vi "Get Public Events.vi"(8 "error in (no error)":errorcluster, 11 "RPI.SenseHat.Actor in":refnum<class "RPI.SenseHat.Actor.lvclass">) -> (0 "error out":errorcluster, 2 "Public Events":T1, 3 "RPI.SenseHat.Actor out":refnum<class "RPI.SenseHat.Actor.lvclass">)   [LabVIEW 2020, in "RPI.SenseHat.Actor.lvlib" / "RPI.SenseHat.Actor.lvclass"]
uses:
  RPI.SenseHat.Actor.lvclass
  Public Events.ctl
  RPI.SenseHat.Joystick/TypeDefs/Joystick.ctl
  RPI.SenseHat.Actor.lvclass/RPI.SenseHat.Actor.ctl
  RPI.SenseHat.Joystick/RPI.SenseHat.Joystick.lvlib
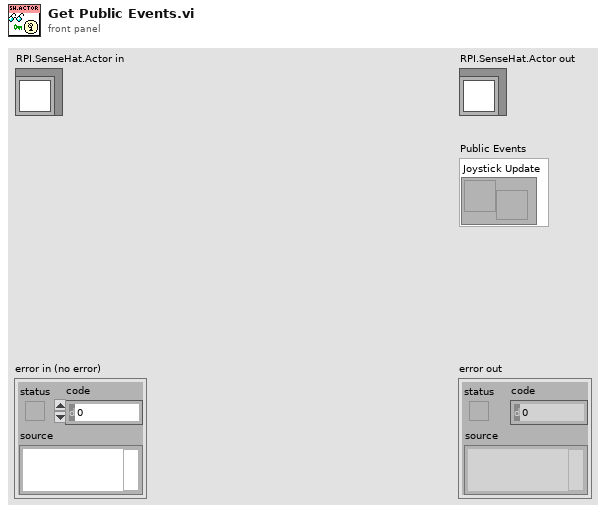
[diagram p1: front panel]
types:
  T1 = typedef "RPI.SenseHat.Actor.lvlib/RPI.SenseHat.Actor.lvclass/Public Events.ctl" = cluster{"Joystick Update":refnum<user-event>}
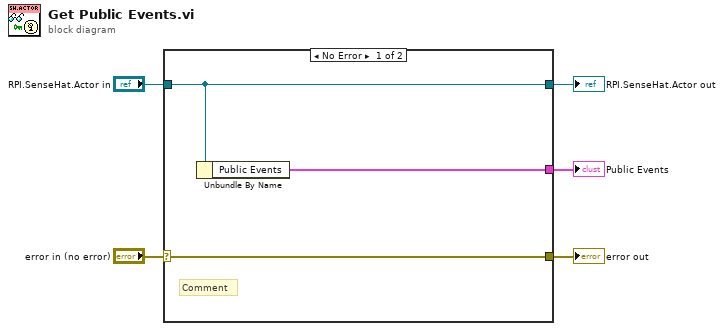
[diagram p0: block diagram]
diagram:
  n1 = case shown="No Error" "error in (no error)" {
    selector: "error in (no error)" -> [w8 w9]
    tunnel: [w8 w9] -> w4
    tunnel: [w7 w10] -> w2
    tunnel: "RPI.SenseHat.Actor in" -> [w7 w10]
    tunnel: [w6 _] -> w1
    frame No Error {
      # "Comment"
      n2 = Unbundle By Name(w7) -> ("Public Events"=w6:T1)
    }
    frame Error {
    }
  }
  "error out" <- w4
  "RPI.SenseHat.Actor out" <- w2
  "Public Events" <- w1
